vi "ZNB data.vi"(8 "error in (no error)":errorcluster, 11 "VISA resource name":refnum<visa-resource-name>) -> (0 "error out":errorcluster, 1 "Real Matrix":T1, 3 "VISA resource name out":refnum<visa-resource-name>)   [LabVIEW 2015]
uses:
  <vilib>/Analysis/Matrix/Datatypes/RealMatrix.ctl
  <instrlib>/Rohde&Schwarz Vector Network Analyzer/Rohde&Schwarz Vector Network Analyzer.lvlib
  <vilib>/Analysis/Matrix/NI_Matrix.lvlib
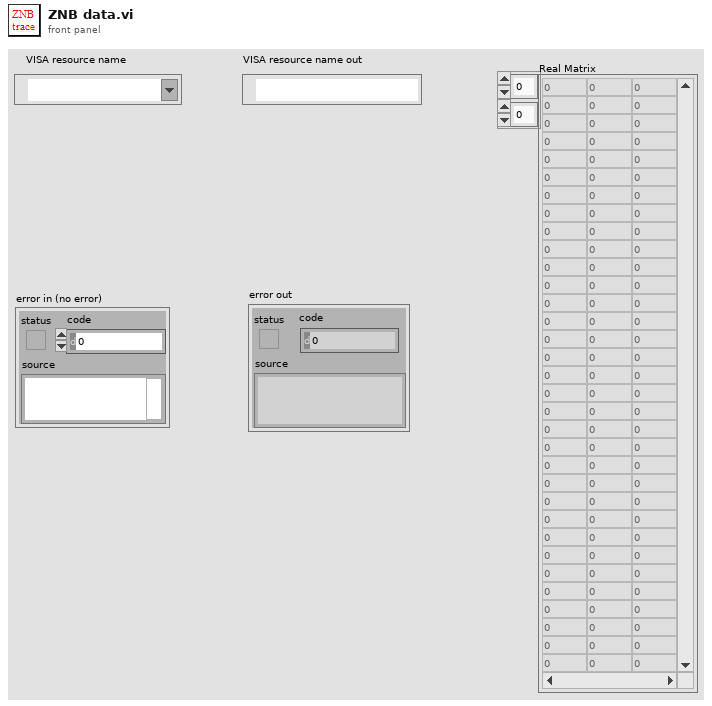
[diagram p1: front panel]
types:
  T1 = typedef "NI_Matrix.lvlib/RealMatrix.ctl" = dbl[][]
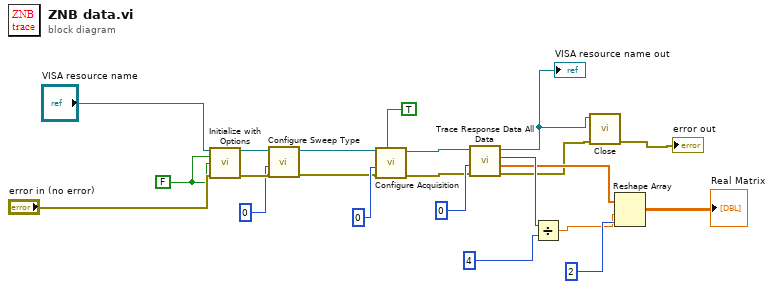
[diagram p0: block diagram]
diagram:
  w13 = FALSE
  n1 = call <instrlib>:"Initialize with Options.vi"("VISA resource name"="VISA resource name", "ID Query (T: Check)"=w13, "Reset (T: Reset)"=w13, "error in (no error)"="error in (no error)") -> ("VISA resource name out"=w6:refnum<visa-resource-name>, "error out"=w7:errorcluster)  [unwired: 10 in]
  n2 = call <instrlib>:"Configure Sweep Type.vi"("error in (no error)"=w7, "Sweep Type (Power)"=0, "VISA resource name"=w6) -> ("error out"=w2:errorcluster, "VISA resource name out"=w1:refnum<visa-resource-name>)  [unwired: 7 in]
  n3 = call <instrlib>:"Configure Acquisition.vi"("Sweep Mode Continuous (F)"=TRUE, "error in (no error)"=w2, "Continuous Sweep Scope (All Channels)"=0, "VISA resource name"=w1) -> ("error out"=w8:errorcluster, "VISA resource name out"=w9:refnum<visa-resource-name>)  [unwired: 6 in]
  n4 = call <instrlib>:"Trace Response Data All Data.vi"("error in (no error)"=w8, "Data Format (Unformatted)"=0, "VISA resource name"=w9) -> ("error out"=w12:errorcluster, "Trace Data"=w18:dbl[], "No of Values"=w19:i32, "VISA resource name out"=w11:refnum<visa-resource-name>)  [unwired: 5 in]
  "VISA resource name out" <- w11
  n5 = Divide(x=w19, y=4) -> (x/y=w17:dbl)
  n6 = call <instrlib>:"Close.vi"("error in (no error)"=w12, "VISA resource name"=w11) -> ("error out"=→"error out":errorcluster)  [unwired: 9 in]
  n7 = Reshape Array(w18, w17, 2) -> (→"Real Matrix":dbl[][])
